vi "format_log_line.vi"(8 "error in (no error)":errorcluster, 9 "timestamp format":string="%^<%Y-%m-%dT%H:%M:%S%3u>TZ", 10 "line format":string="{{timestamp}} | {{level}} | {{context}} | {{message}}", 11 "message":T1 {"level" items=["OFF"=0, "FATAL"=100, "ERROR"=200, "WARN"=300, "INFO"=400, "DEBUG"=500, "TRACE"=600, "ALL"=65535]}) -> (0 "error out":errorcluster, 3 "formatted log line":string)   [LabVIEW 2019, in "File Log Provider.lvclass"]
uses:
  Queue Log Provider/impl/log_message.ctl
  Log Service/public/level.ctl
  File Log Provider.lvclass
  Log Service/Log Service.lvclass
  Queue Log Provider/Queue Log Provider.lvclass
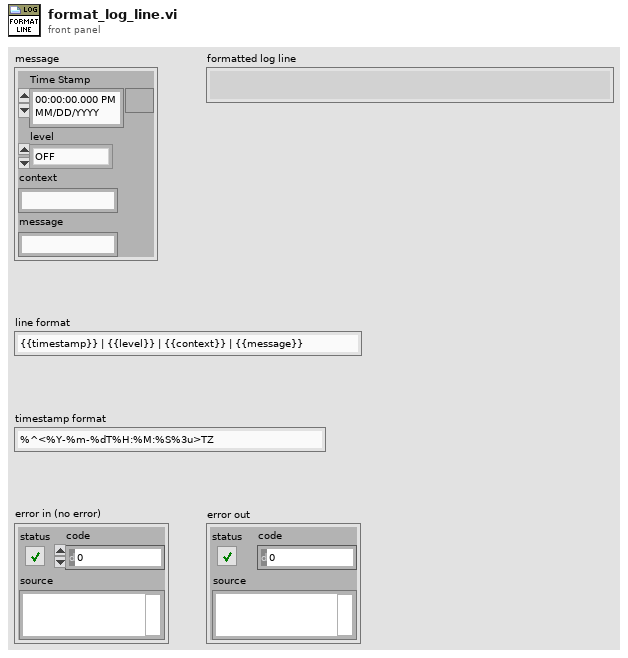
[diagram p1: front panel]
types:
  T1 = typedef "Queue Log Provider.lvclass/log_message.ctl" = cluster{"Time Stamp":timestamp, "level":T2, "context":string, "message":string}
  T2 = typedef "Utility API.lvlib/Log Service.lvclass/level.ctl" = u16
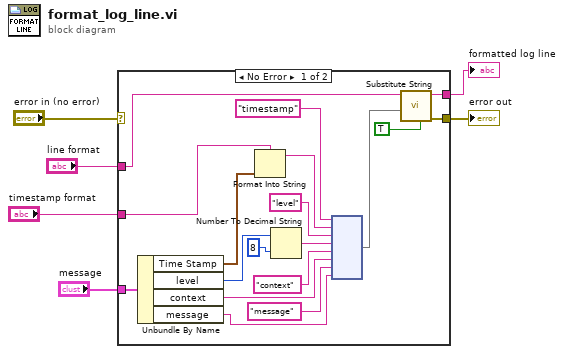
[diagram p0: block diagram]
diagram:
  n1 = case shown="No Error" "error in (no error)" {
    selector: "error in (no error)" -> [_ w25]
    tunnel: [w24 w25] -> w6
    tunnel: [w23 _] -> w5
    tunnel: "line format" -> [w22 _]
    tunnel: "timestamp format" -> [w21 _]
    tunnel: "message" -> [w20 _]
    frame No Error {
      n2 = Unbundle By Name(w20) -> ("Time Stamp"=w18:timestamp, "level"=w15:T2, "context"=w11:string, "message"=w9:string)
      n3 = Format Into String(format string=w21, w18) -> (resulting string=w17:string)  [unwired: 2 in, 1 out]
      n4 = Number To Decimal String(number=w15, width (-)=i16 8) -> (decimal integer string=w13:string)
      n5 = node("timestamp" ("key"), w17, "level" ("key"), w13, "context" ("key"), w11, "message" ("key"), w9) -> (w8:map{string, string})
      n6 = call "Substitute String.vi"("use cached delimeter pattern data? (F)"=TRUE, "substitutions"=w8, "input string"=w22) -> ("error out"=w24:errorcluster, "output string"=w23:string)  [unwired: 7 in]
    }
    frame Error {
    }
  }
  "error out" <- w6
  "formatted log line" <- w5
